vi "Initiate Generation Core.vi"(8 "error in (no error)":errorcluster, 11 "IVI_Fgen in":refnum<class "IVI_Fgen.lvclass">) -> (0 "error out":errorcluster, 3 "IVI_Fgen out":refnum<class "IVI_Fgen.lvclass">)   [LabVIEW 2016, in "IVI_Fgen.lvlib" / "IVI_Fgen.lvclass"]
doc: "This VI initiates signal generation. If the function generator is in the Configuration State, this VI moves the function generator to the Output Generation State. If the function generator is already in the Output Generation State, this VI does nothing.\n\nThe instrument is in the Generation State after you call the IviFgen Initialize, IviFgen Initialize With Options, or IviFgen Reset VIs. You can configure the output of the function generator regardless of whether function generator is in the Configuration State or the Generation State. This means that you are required to call the IviFgen Initiate Generation VI only if you abort signal generation by calling the IviFgen Abort Generation VI. \n\nMany function generators constantly generate an output signal, and do not require you to initiate signal generation. If a function generator is always outputting the currently configured signal, this VI does nothing.\n\nYou are not required to call the IviFgen Initiate Generation and IviFgen Abort Generation VIs. Whether you choose to call these VIs in an application program has no impact on interchangeability. You can choose to use these VIs if you want to optimize your application for instruments that exhibit increased performance when output configuration is performed while the instrument is not generating a signal.\n\nThis VI disables extensions that have not been set by the user under the following conditions:\n\n(1) If you have not set the value of any property in the IviFgenModulateAM extension on a channel, this VI sets the IviFgen>>Amplitude Modulation Attributes>>AM Enabled [AM] property to FALSE for that channel.\n\n(2) If you have not set the value of any property in the IviFgenModulateFM extension on a channel, this VI sets the IviFgen>>Frequency Modulation Attributes>>FM Enabled [FM] property to FALSE for that channel.\n\nNotes:\n\n(1) This VI does not normally check the instrument status. Typically, you call this VI only in a sequence of calls to other low-level driver functions. The sequence performs one operation. You use the low-level VIs to optimize one or more aspects of interaction with the instrument. If you want to check the instrument status, call the IviFgen Error-Query VI at the conclusion of the sequence.\n\n(2) This VI performs interchangeability checking when the IviFgen>>Inherent IVI Settings>>User Options>>Interchange Check property is set to TRUE. If the IviFgen>>Inherent IVI Settings>>User Options>>Spy property is set to TRUE, you use the NI I/O Trace utility to view interchangeability warnings. You use the IviFgen Get Next Interchange Warning VI to retrieve interchangeability warnings when the IviFgen>>Inherent IVI Settings>>User Options>>Spy property is set to FALSE. For more information about interchangeability checking, refer to the help text for the IviFgen>>Inherent IVI Settings>>User Options>>Interchange Check property."
uses:
  IVI_Fgen.lvclass
  IVI_Fgen.lvclass/IVI_Fgen.ctl
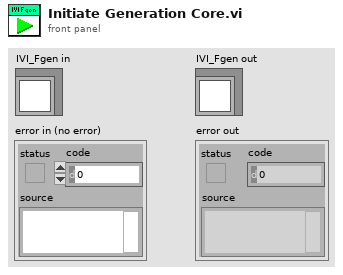
[diagram p1: front panel]
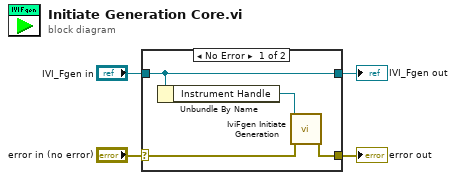
[diagram p0: block diagram]
diagram:
  n1 = case shown="No Error" "error in (no error)" {
    selector: "error in (no error)" -> [w6 w10]
    tunnel: [w5 w10] -> w3
    tunnel: [w8 w9] -> w1
    tunnel: "IVI_Fgen in" -> [w8 w9]
    frame No Error {
      n2 = Unbundle By Name(w8) -> ("Instrument Handle"=w7:refnum<k15>)
      n3 = call <vilib>:"IviFgen Initiate Generation.vi"("error in (no error)"=w6, "instrument handle"=w7) -> ("error out"=w5:errorcluster)  [unwired: 8 in, 1 out]
    }
    frame Error {
    }
  }
  "error out" <- w3
  "IVI_Fgen out" <- w1
